vi "AutoMoveSubVI.vi"() -> ()   [LabVIEW 2010]
uses:
  <vilib>/NXT/Subs/MotorXNode.DC Motor Type.ctl
  <vilib>/NXT/Subs/LVHSConnector.ctl
  <vilib>/NXT/HiTechnic/HiTechnic Controls/HiTechnic Port.ctl
  <vilib>/NXT/Block Support/NXT_InputPort.ctl
  <vilib>/NXT/NXTIO Xnodes/NXTIOXNode/NXTIO.xnode
  <vilib>/NXT/Subs/MotorXNode.2DCMotor.ctl
  <vilib>/NXT/NXTIO Xnodes/NXTIONodeSubVIs/TETRIX IO Move DC Motors.vi
panel:
  in  "index":i32
  in  "NXT 2":T1
  in  "Power/Speed 1":i8
  out "NXT":T1
  in  "DC Motor":T3
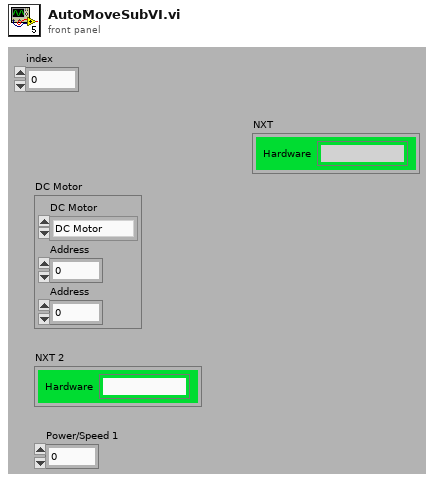
[diagram p1: front panel]
types:
  T1 = typedef "LVHSConnector.ctl" = cluster{"Hardware":string, "Flattened String":string}
  T2 = typedef "MotorXNode.DC Motor Type.ctl" = enum16{"DC Motor"}
  T3 = cluster{"DC Motor":T2, "Address":i16, "Address":i16}
  T4 = typedef "HiTechnic Port.ctl" = cluster{"Port":T5, "MUX Port":u8}
  T5 = typedef "NXT_InputPort.ctl" = u8
  T6 = cluster{"Direction (0-9)":i16, "Signal Strength (Array)":u8[]}
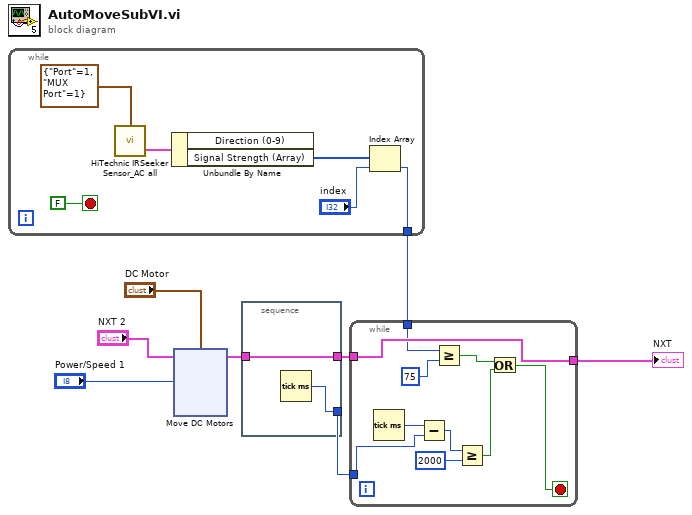
[diagram p0: block diagram]
diagram:
  n1 = while {
    tunnel: [w10] -> w1
    stop <- FALSE stop-if-true
    n2 = call <vilib>:"HiTechnic IRSeeker Sensor_AC all.vi"("Port/MUX"=T4 {"Port"=1, "MUX Port"=1}) -> ("All Info"=w13:T6)  [unwired: 2 in, 1 out]
    n3 = Unbundle By Name(w13) -> ("Signal Strength (Array)"=w12:u8[])  [unwired: 1 out]
    n4 = Index Array(array=w12, index="index") -> (element=w10:u8)
  }
  n5 = xnode "Move DC Motors"("Power/Speed 1"="Power/Speed 1", "Motors"="DC Motor", "NXT"="NXT 2") -> ("NXT"=w6:T1)  [unwired: 1 in]
  n6 = stacked-sequence {
    tunnel: [w16] -> w5
    tunnel: w6 -> [w15]
    tunnel: [w15] -> w3
    frame #0 {
      n7 = Tick Count (ms)() -> (millisecond timer value=w16:u32)
    }
  }
  n8 = while {
    tunnel: w5 -> [w26]
    tunnel: w3 -> [w19]
    tunnel: [w19] -> w2
    tunnel: w1 -> [w18]
    stop <- w17 stop-if-true
    n9 = Tick Count (ms)() -> (millisecond timer value=w24:u32)
    n10 = Subtract(x=w24, y=w26) -> (x-y=w23:u32)
    n11 = Greater Or Equal?(x=w18, y=u8 75) -> (x >= y?=w21:bool)
    n12 = Greater Or Equal?(x=w23, y=u32 2000) -> (x >= y?=w20:bool)
    n13 = Or(x=w21, y=w20) -> (x .or. y?=w17:bool)
  }
  "NXT" <- w2
